vi "Unix vs LabVIEW epoch.vi"() -> (0 "seconds from 1904-01-01 to 1970-01-01":i64)   [LabVIEW 2020, in "NI_SFTP.lvlib" / "File Attributes.lvclass"]
uses:
  <vilib>/net/SFTP/File Attributes/File Attributes.lvclass
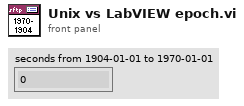
[diagram p1: front panel]
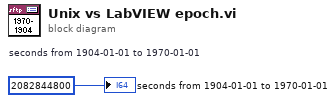
[diagram p0: block diagram]
diagram:
  w1 = i64 2082844800  # seconds from 1904-01-01 to 1970-01-01
  "seconds from 1904-01-01 to 1970-01-01" <- w1
